vi "UIStep Execte UI.vi"(8 "error in (no error)":errorcluster, 10 "Project Path":path, 11 "UI Setting":T1={"Embedded"=FALSE, "Size"=enum."Small", "Title"="", "Content"="", "Text Style"={"Font"="", "Size"=0.0, "Justification"=1, "TextColor"=0, "BGColor"=0, "Bold"=FALSE}, "Buttons"={"Button1"={"Label"="", "Size"=0.0, "TextColor"=0, "BGColor"=0, "Bold"=FALSE}, "Button2"={"Label"="", "Size"=0.0, "TextColor"=0, "BGColor"=0, "Bold"=FALSE}}, "Image"=path "", "Enable Input"=FALSE, "Input Validation"=""} {"Text Style"."Justification" items=["Left", "Center", "Right"]}) -> (0 "error out":errorcluster, 3 "Output Values":cluster{"Name":string, "Variant Data":variant}[](array[cluster]))   [LabVIEW 2015, in "UIStep.lvclass"]
uses:
  UIStep.lvclass
  UI_STATE_TYPE_DEF.ctl
  <vilib>/Utility/miscctls.llb/LVKeyTypeDef.ctl
  <vilib>/event_ctls.llb/eventvkey.ctl
  <vilib>/ErrorRing/Error Ring.xnode
panel:
  in  "Input":string
  out "Image":picture
  in  "Button2":bool
  in  "Button1":bool
  out "Content":string
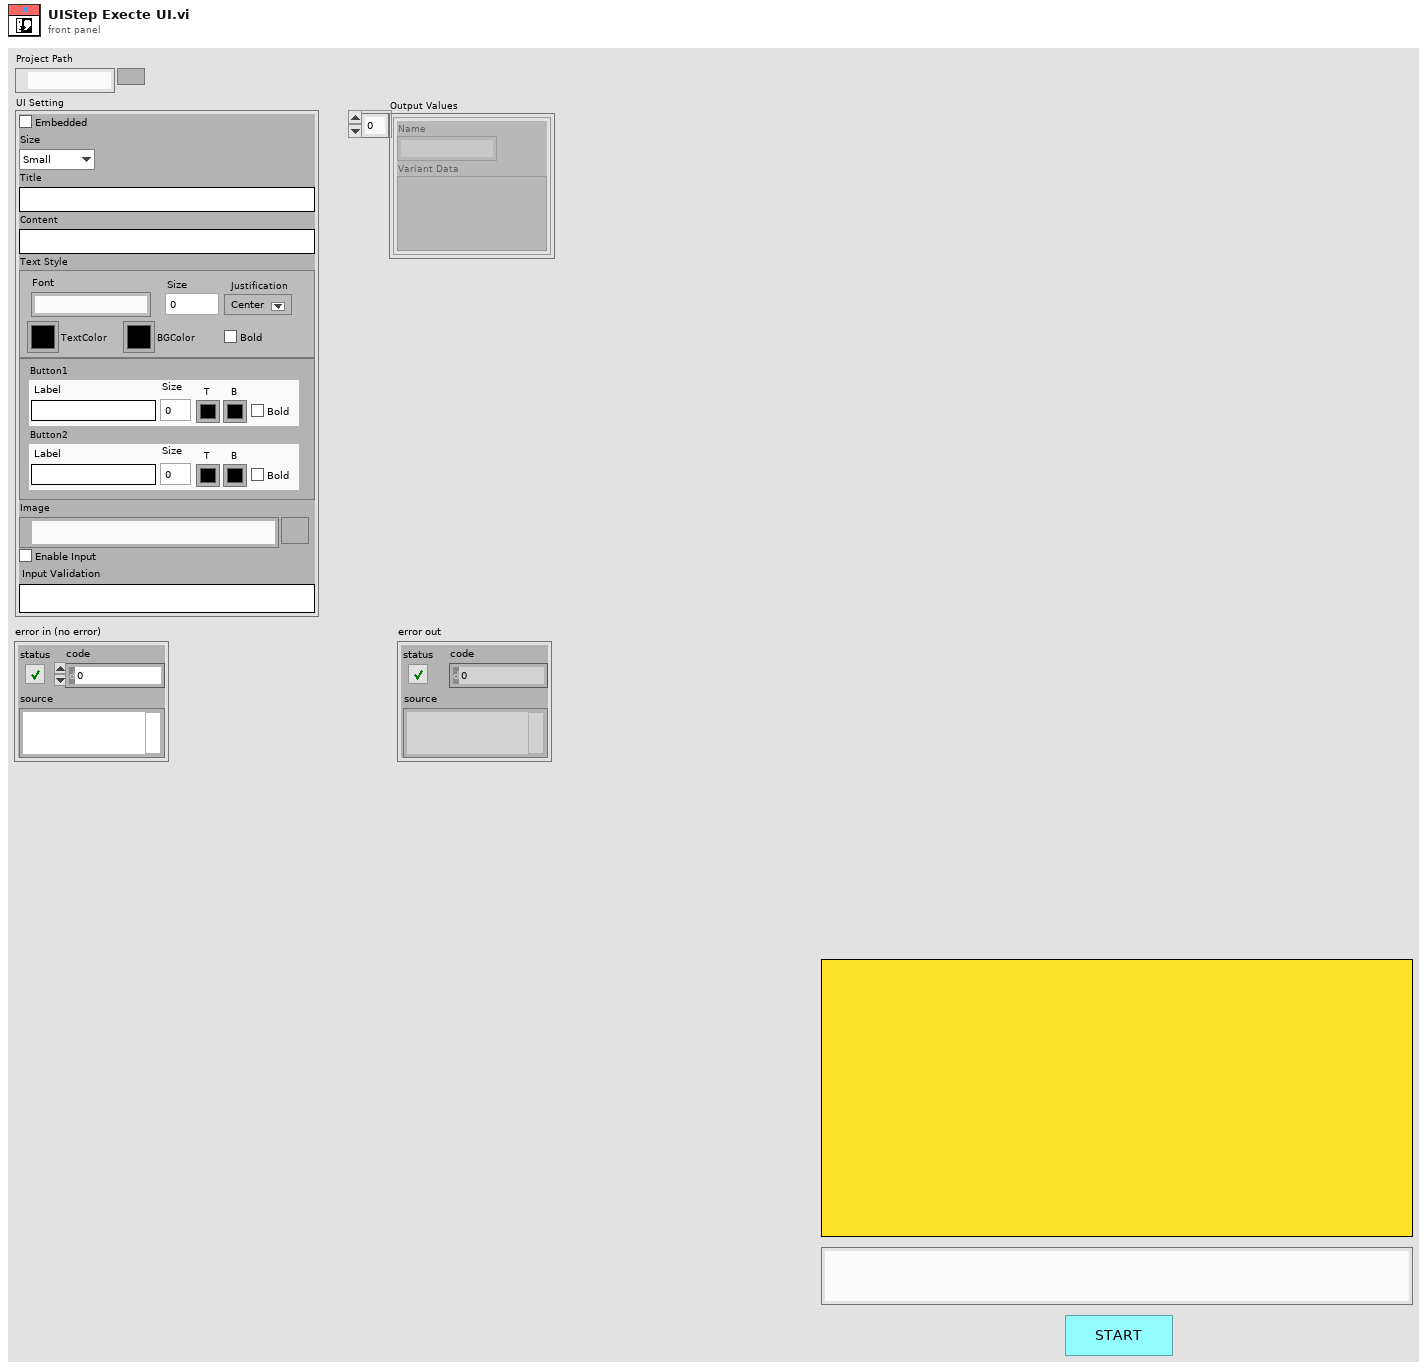
[diagram p1: front panel]
types:
  T1 = cluster{"Embedded":bool, "Size":enum16{"Small", "Middle", "Big"}, "Title":string, "Content":string, "Text Style":cluster{"Font":string, "Size":dbl, "Justification":u16, "TextColor":u32, "BGColor":u32, "Bold":bool}, "Buttons":cluster{"Button1":cluster{"Label":string, "Size":dbl, "TextColor":u32, "BGColor":u32, "Bold":bool}, "Button2":cluster{"Label":string, "Size":dbl, "TextColor":u32, "BGColor":u32, "Bold":bool}}, "Image":path, "Enable Input":bool, "Input Validation":string}
  T2 = cluster{"VI":refnum<vi>, "Content":refnum<vi>, "Input":refnum<vi>, "Image":refnum<vi>, "Button1":refnum<vi>, "Button2":refnum<vi>}
  T3 = typedef "UIStep.lvclass/UI_STATE_TYPE_DEF.ctl" = enum16{"INIT", "END", "UI_LOOP"}
  T4 = enum32{"Invalid", "Standard", "Closed", "Hidden", "Minimized", "Maximized"}
  T5 = typedef "LVKeyTypeDef.ctl" = cluster{"Focus":bool, "Control":bool, "Shift":bool, "Key":string}
  T6 = typedef "eventvkey.ctl" = enum16{"ASCII", "Enter", "Return", "Shift", "Ctrl", "Alt", "Cmd", "Opt", "Caps", "NumLock", "Clear", "Break", "Up", "Down", "Left", "Right", "Insert", "Delete", "Home", "End", "PageUp", "PageDown", "Escape", "Help", "Pause", "ScrollLock", "F1", "F2", "F3", "F4", "F5", "F6", "F7", "F8", "F9", "F10", "F11", "F12", "F13", "F14", "F15", "F16", "F17", "F18", "F19", "F20", "F21", "F22", "F23", "F24", "Play", "VolumeUp", "VolumeDown", "Mute", "Two Byte Char"}
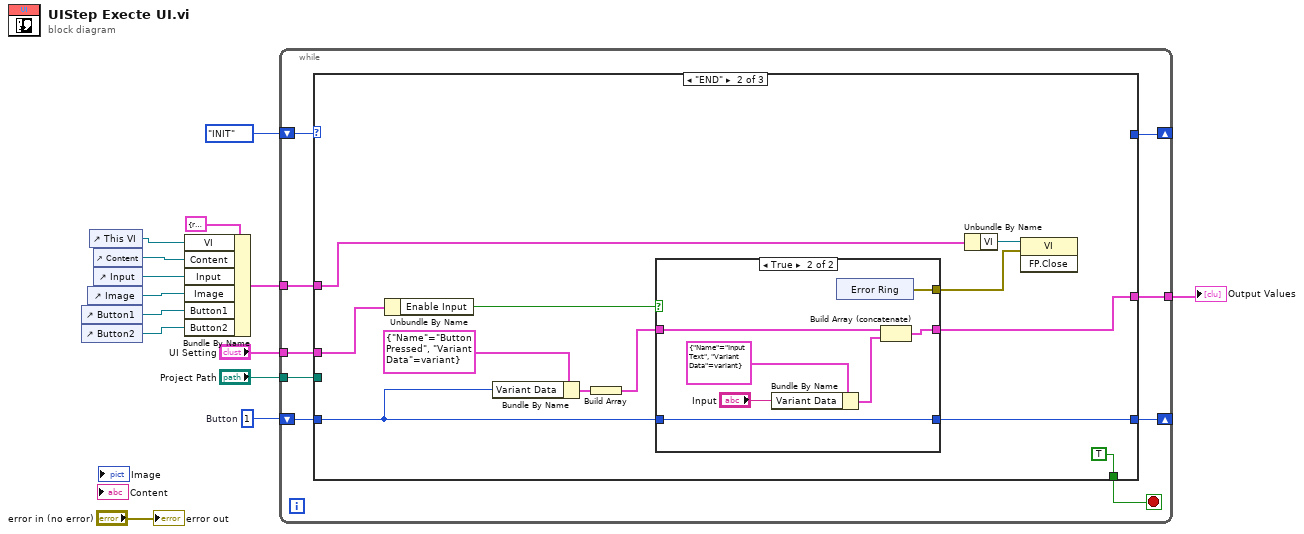
[diagram p0: block diagram]
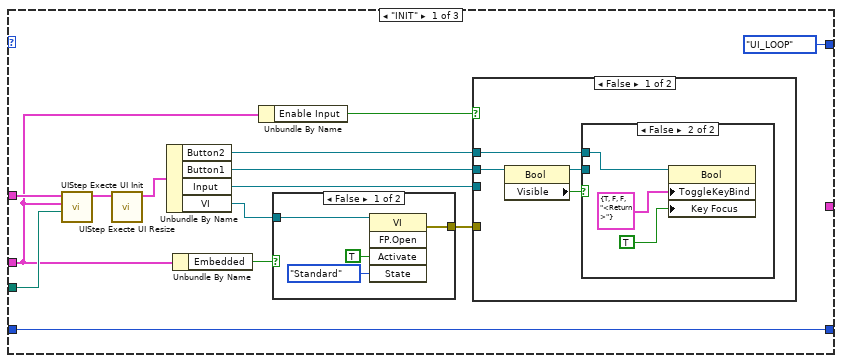
[diagram p2: hidden frame]
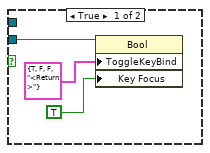
[diagram p4: hidden frame]
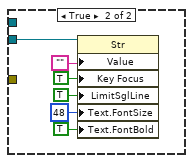
[diagram p5: hidden frame]
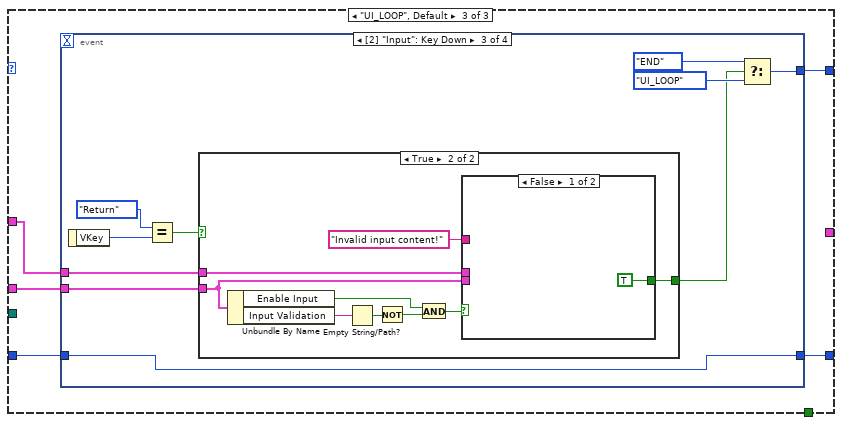
[diagram p7: hidden frame]
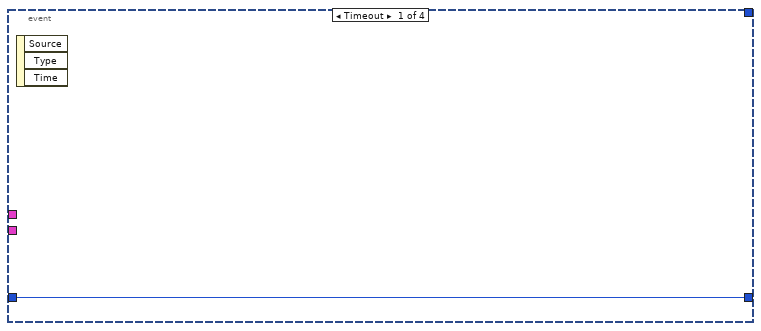
[diagram p8: hidden frame]
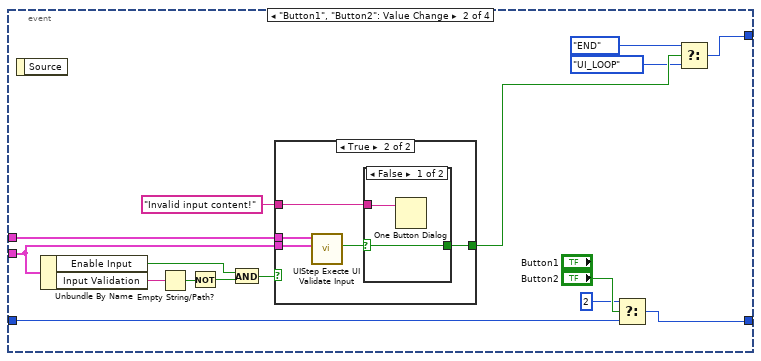
[diagram p9: hidden frame]
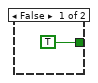
[diagram p10: hidden frame]
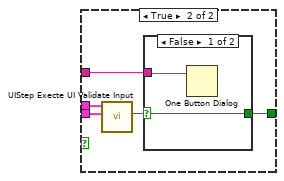
[diagram p13: hidden frame]
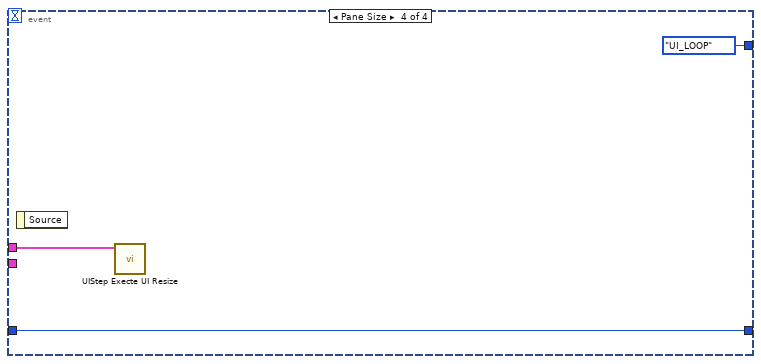
[diagram p15: hidden frame]
diagram:
  w1 = 1  # Button
  n1 = control-ref of="Button1"() -> (w9:refnum<vi>)
  n2 = control-ref of="Button2"() -> (w8:refnum<vi>)
  n3 = control-ref of="Image"() -> (w10:refnum<vi>)
  n4 = control-ref of="This VI"() -> (w6:refnum<vi>)
  n5 = control-ref of="Content"() -> (w12:refnum<vi>)
  n6 = control-ref of="Input"() -> (w11:refnum<vi>)
  n7 = Bundle By Name(cluster=T2 {"VI"=refnum, "Content"=refnum, "Input"=refnum, "Image"=refnum, "Button1"=refnum, "Button2"=refnum}, "VI"=w6, "Content"=w12, "Input"=w11, "Image"=w10, "Button1"=w9, "Button2"=w8) -> (w7:T2)
  n8 = while {
    shift-right: [w21] -> _
    shift-left: UI_STATE_TYPE_DEF."INIT" -> [w23]
    tunnel: w7 -> [w20]
    tunnel: "UI Setting" -> [w19]
    tunnel: "Project Path" -> [w18]
    tunnel: [w17] -> w4
    shift-right: [w15] -> _
    shift-left: w1 -> [w16]
    stop <- w22 stop-if-true
    n9 = case shown="\"END\"" w23 {
      tunnel: [_ TRUE _] -> w22
      tunnel: [UI_STATE_TYPE_DEF."UI_LOOP" _ w84] -> w21
      tunnel: w20 -> [w35 w67 w83]
      tunnel: w19 -> [w27 w65 w82]
      tunnel: w18 -> [w36 _ _]
      tunnel: [_ w60 _] -> w17
      tunnel: w16 -> [w28 w59 w81]
      tunnel: [w28 w61 w80] -> w15
      frame "INIT" {
        n10 = call "UIStep Execte UI Init.vi"("Project Path"=w36, "UI Setting"=w27, "UI Control"=w35) -> ("UI Control out"=w34:T2)  [unwired: 8 in]
        n11 = call "UIStep Execte UI Resize.vi"("UI Control"=w34) -> ("UI Control out"=w33:T2)  [unwired: 10 in]
        n12 = Unbundle By Name(w33) -> ("Button2"=w24:refnum<vi>, "Button1"=w25:refnum<vi>, "Input"=w29:refnum<vi>, "VI"=w32:refnum<vi>)
        n13 = Unbundle By Name(w27) -> ("Embedded"=w26:bool)
        n14 = Unbundle By Name(w27) -> ("Enable Input"=w31:bool)
        n15 = case shown="False" w26 {
          tunnel: w32 -> [w41 _]
          tunnel: [w38 _] -> w30
          frame False {
            n16 = invoke class="VI" method="FP.Open"(reference=w41, "Activate"=TRUE ("Activate?"), "State"=T4."Standard") -> (error out=w38:errorcluster)  [unwired: 2 in, 4 out]
          }
          frame True {
          }
        }
        n17 = case shown="False" w31 {
          tunnel: w30 -> [_ _]
          tunnel: w29 -> [_ w57]
          tunnel: w25 -> [w45 _]
          tunnel: w24 -> [w42 _]
          frame False {
            n18 = property class="Bool"(reference=w45) -> (reference out=w43:refnum<vi>, "Visible"=w44:bool)  [unwired: 1 in, 1 out]
            n19 = case shown="False" w44 {
              tunnel: w43 -> [w48 _]
              tunnel: w42 -> [_ w49]
              frame True {
                n20 = property class="Bool"(reference=w48, "ToggleKeyBind"=T5 {"Focus"=TRUE, "Control"=FALSE, "Shift"=FALSE, "Key"="<Return>"} ("Toggle Key Binding"), "Key Focus"=TRUE) -> ()  [unwired: 1 in, 2 out]
              }
              frame False {
                n21 = property class="Bool"(reference=w49, "ToggleKeyBind"=T5 {"Focus"=TRUE, "Control"=FALSE, "Shift"=FALSE, "Key"="<Return>"} ("Toggle Key Binding"), "Key Focus"=TRUE) -> ()  [unwired: 1 in, 2 out]
              }
            }
          }
          frame True {
            n22 = property class="Str"(reference=w57, "Value"="", "Key Focus"=TRUE, "LimitSglLine"=TRUE ("Limit To Single Line?"), "Text.FontSize"=u32 48 ("Text.Font:Size"), "Text.FontBold"=TRUE ("Text.Font:Bold")) -> ()  [unwired: 1 in, 2 out]
          }
        }
      }
      frame "END" {
        n23 = Unbundle By Name(w65) -> ("Enable Input"=w64:bool)
        n24 = Bundle By Name(cluster=cluster{"Name":string, "Variant Data":variant} {"Name"="Button Pressed", "Variant Data"=variant}, "Variant Data"=w59) -> (w63:cluster{"Name":string, "Variant Data":variant})
        n25 = Build Array(w63) -> (w62:cluster{"Name":string, "Variant Data":variant}[])
        n26 = case shown="True" w64 {
          tunnel: w62 -> [w70 w76]
          tunnel: w59 -> [w71 w78]
          tunnel: [w71 w78] -> w61
          tunnel: [w70 w74] -> w60
          tunnel: [_ w73] -> w58
          frame False {
          }
          frame True {
            n27 = Bundle By Name(cluster=cluster{"Name":string, "Variant Data":variant} {"Name"="Input Text", "Variant Data"=variant}, "Variant Data"="Input") -> (w75:cluster{"Name":string, "Variant Data":variant})
            n28 = xnode "Error Ring"() -> ("error out"=w73:errorcluster)
            n29 = Build Array (concatenate)(w76, w75) -> (w74:cluster{"Name":string, "Variant Data":variant}[])
          }
        }
        n30 = Unbundle By Name(w67) -> ("VI"=w68:refnum<vi>)
        n31 = invoke class="VI" method="FP.Close"(reference=w68, error in=w58) -> ()  [unwired: 1 in, 3 out]
      }
      frame "UI_LOOP", Default {
        n32 = event shown="[2] \"Input\": Key Down" {
          selector: _ -> [_ _ _ _]
          dyn-events: _ -> [_ _ _ _]
          timeout: _ -> [_ _ _ _]
          tunnel: [_ w91 w116 UI_STATE_TYPE_DEF."UI_LOOP"] -> w84
          tunnel: w83 -> [_ w101 w120 w140]
          tunnel: w82 -> [_ w95 w119 _]
          tunnel: w81 -> [w85 w87 w111 w139]
          tunnel: [w85 w86 w111 w139] -> w80
          event Timeout {
            n33 = event-data() -> ()  [unwired: 1 in, 3 out]
          }
          event "Button1", "Button2": Value Change {
            n34 = event-data() -> ()  [unwired: 1 in, 1 out]
            n35 = Unbundle By Name(w95) -> ("Enable Input"=w97:bool, "Input Validation"=w100:string)
            n36 = Empty String/Path?(string/path=w100) -> (empty?=w99:bool)
            n37 = Not(x=w99) -> (.not. x?=w98:bool)
            n38 = And(x=w97, y=w98) -> (x .and. y?=w96:bool)
            n39 = case shown="True" w96 {
              tunnel: w101 -> [_ w107]
              tunnel: w95 -> [_ w106]
              tunnel: [TRUE w104] -> w94
              tunnel: "Invalid input content!" ("message") -> [_ w103]
              frame False {
              }
              frame True {
                n40 = call "UIStep Execte UI Validate Input.vi"("UI Setting"=w106, "UI Control"=w107) -> ("Valid out"=w105:bool)  [unwired: 8 in, 1 out]
                n41 = case shown="False" w105 {
                  selector: w105 -> [w109 w110]
                  tunnel: [w109 w110] -> w104
                  tunnel: w103 -> [w108 _]
                  frame False {
                    n42 = One Button Dialog(message=w108) -> ()  [unwired: 1 in, 1 out]
                  }
                  frame True {
                  }
                }
              }
            }
            n43 = Select(t=2, s="Button2", f=w87) -> (s? t:f=w86:i32)
            n44 = Select(t=UI_STATE_TYPE_DEF."END", s=w94, f=UI_STATE_TYPE_DEF."UI_LOOP") -> (s? t:f=w91:T3)
          }
          event "Input": Key Down {
            n45 = event-data() -> ("VKey"=w114:T6)  [unwired: 1 in]
            n46 = Equal?(x=eventvkey."Return" ("VKey"), y=w114) -> (x = y?=w112:bool)
            n47 = case shown="True" w112 {
              tunnel: w120 -> [_ w123]
              tunnel: w119 -> [_ w122]
              tunnel: [_ w121] -> w115
              frame False {
              }
              frame True {
                n48 = Unbundle By Name(w122) -> ("Enable Input"=w126:bool, "Input Validation"=w129:string)
                n49 = Empty String/Path?(string/path=w129) -> (empty?=w128:bool)
                n50 = Not(x=w128) -> (.not. x?=w127:bool)
                n51 = And(x=w126, y=w127) -> (x .and. y?=w125:bool)
                n52 = case shown="False" w125 {
                  tunnel: w123 -> [_ w135]
                  tunnel: w122 -> [_ w134]
                  tunnel: [TRUE w132] -> w121
                  tunnel: "Invalid input content!" ("message") -> [_ w131]
                  frame False {
                  }
                  frame True {
                    n53 = call "UIStep Execte UI Validate Input.vi"("UI Setting"=w134, "UI Control"=w135) -> ("Valid out"=w133:bool)  [unwired: 8 in, 1 out]
                    n54 = case shown="False" w133 {
                      selector: w133 -> [w137 w138]
                      tunnel: [w137 w138] -> w132
                      tunnel: w131 -> [w136 _]
                      frame False {
                        n55 = One Button Dialog(message=w136) -> ()  [unwired: 1 in, 1 out]
                      }
                      frame True {
                      }
                    }
                  }
                }
              }
            }
            n56 = Select(t=UI_STATE_TYPE_DEF."END", s=w115, f=UI_STATE_TYPE_DEF."UI_LOOP") -> (s? t:f=w116:T3)
          }
          event Pane Size {
            n57 = event-data() -> ()  [unwired: 1 in, 1 out]
            n58 = call "UIStep Execte UI Resize.vi"("UI Control"=w140) -> ()  [unwired: 10 in, 1 out]
          }
        }
      }
    }
  }
  "Output Values" <- w4
  "error out" <- "error in (no error)"
